vi "demo.vi"() -> ()   [LabVIEW 2017]
panel:
  out "z 4":dbl
  out "y 4":dbl
  out "x 4":dbl
  out "z 3":dbl
  out "y 3":dbl
  out "x 3":dbl
  out "z 2":dbl
  out "y 2":dbl
  out "x 2":dbl
  out "rv 2":dbl
  out "cx 3":dbl
  out "cy 3":dbl
  out "cz 3":dbl
  out "vx 3":dbl
  out "vy 3":dbl
  out "vz 3":dbl
  out "cx 2":dbl
  out "cy 2":dbl
  out "cz 2":dbl
  out "vx 2":dbl
  out "vy 2":dbl
  out "vz 2":dbl
  out "vz":dbl
  out "vy":dbl
  out "vx":dbl
  out "cz":dbl
  out "cy":dbl
  out "cx":dbl
  out "gap speed":dbl
  out "gap":dbl
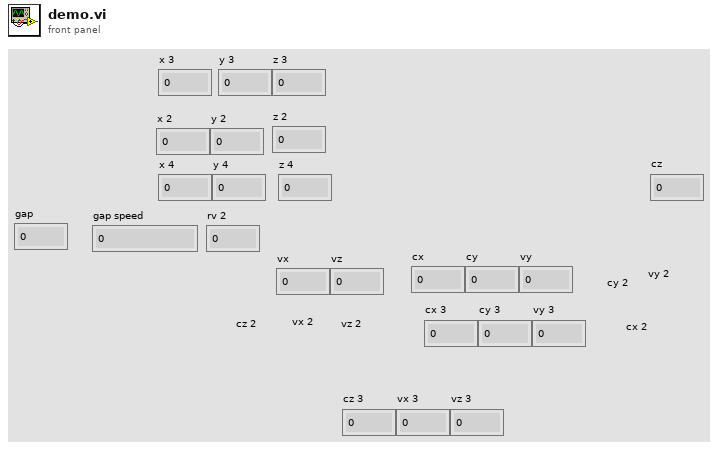
[diagram p1: front panel]
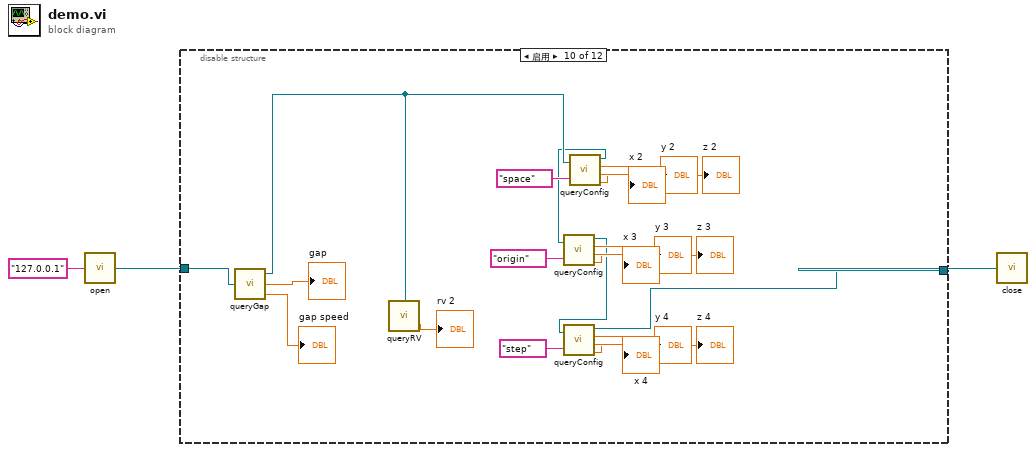
[diagram p0: block diagram]
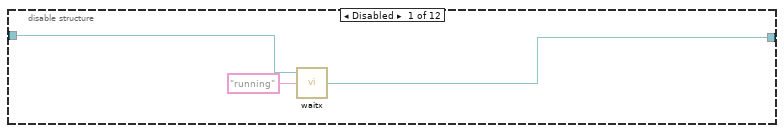
[diagram p2: hidden frame]
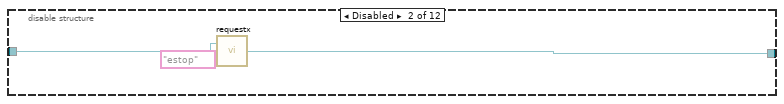
[diagram p3: hidden frame]
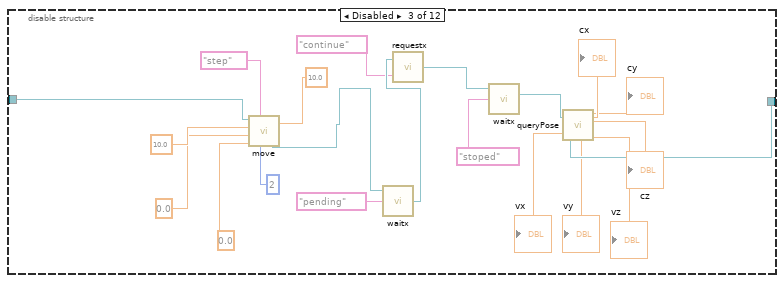
[diagram p4: hidden frame]
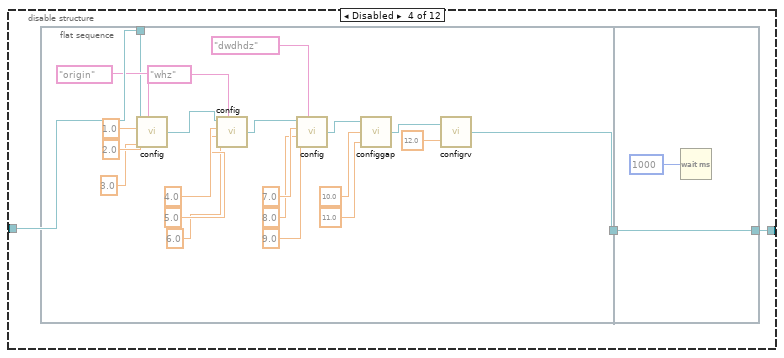
[diagram p5: hidden frame]
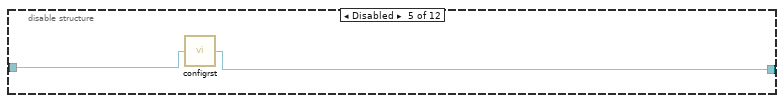
[diagram p6: hidden frame]
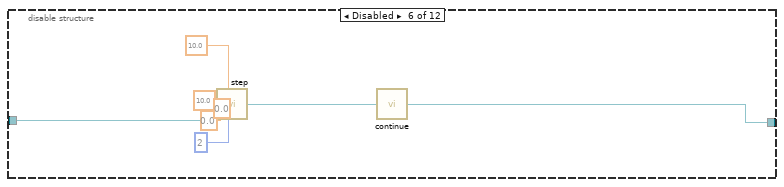
[diagram p7: hidden frame]
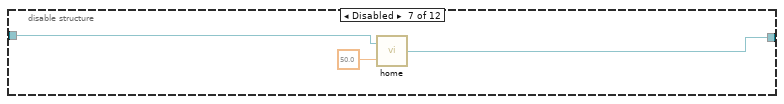
[diagram p8: hidden frame]
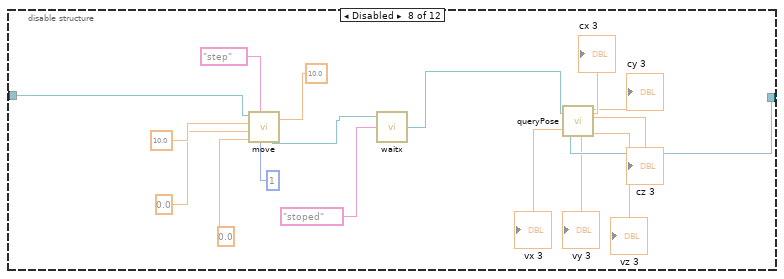
[diagram p9: hidden frame]
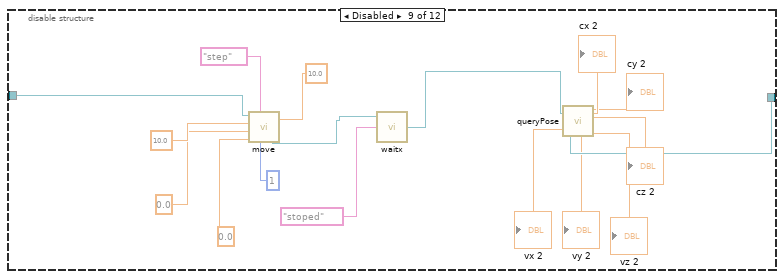
[diagram p10: hidden frame]
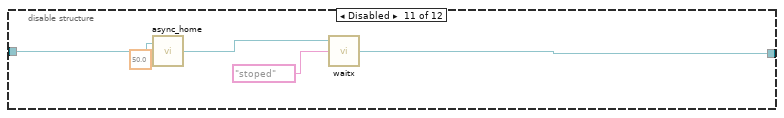
[diagram p11: hidden frame]
diagram:
  n1 = call "open.vi"("地址"="127.0.0.1") -> ("连接ID"=w2:refnum<k5>)
  n2 = disable-structure shown="启用" {
    disable-tunnel: w2 -> [w5 w9 w30 w33 w58 w66 w69 w86 w103 w123 w128 _]
    disable-tunnel: [w4 w7 w18 w32 w57 w59 w67 w73 w90 w104 w124 _] -> w1
    frame Disabled {
      n3 = call "waitx.vi"("String Value"="running", "连接ID"=w5) -> ("连接ID 2"=w4:refnum<k5>)  [unwired: 1 in]
    }
    frame Disabled {
      n4 = call "requestx.vi"("cmd"="estop" ("String"), "连接ID"=w9) -> ("连接ID输出"=w7:refnum<k5>)
    }
    frame Disabled {
      n5 = call "move.vi"("v"=10.0, "n"=2, "String"="step", "z"=0.0 ("zin"), "y"=0.0 ("yin"), "x"=10.0 ("xin"), "连接ID"=w30) -> ("连接ID输出"=w14:refnum<k5>)
      n6 = call "waitx.vi"("String Value"="pending", "连接ID"=w14) -> ("连接ID 2"=w12:refnum<k5>)  [unwired: 1 in]
      n7 = call "requestx.vi"("cmd"="continue" ("String"), "连接ID"=w12) -> ("连接ID输出"=w10:refnum<k5>)
      n8 = call "waitx.vi"("String Value"="stoped", "连接ID"=w10) -> ("连接ID 2"=w22:refnum<k5>)  [unwired: 1 in]
      n9 = call "queryPose.vi"("连接ID"=w22) -> ("连接ID输出"=w18:refnum<k5>, "x"=→"cx":dbl, "vx"=→"vx":dbl, "y"=→"cy":dbl, "z"=→"cz":dbl, "vy"=→"vy":dbl, "vz"=→"vz":dbl)
    }
    frame Disabled {
      n10 = flat-sequence {
        tunnel: w33 -> [w42]
        tunnel: [w37] -> w31
        tunnel: [w56] -> w32
        tunnel: w31 -> [w56]
        frame #0 {
          n11 = call "config.vi"("连接ID"=w42, "x"=1.0, "y"=2.0, "z"=3.0, "item"="origin" ("String")) -> ("连接ID输出"=w36:refnum<k5>)
          n12 = call "config.vi"("连接ID"=w36, "x"=4.0, "y"=5.0, "z"=6.0, "item"="whz" ("String")) -> ("连接ID输出"=w35:refnum<k5>)
          n13 = call "config.vi"("连接ID"=w35, "x"=7.0, "y"=8.0, "z"=9.0, "item"="dwdhdz" ("String")) -> ("连接ID输出"=w34:refnum<k5>)
          n14 = call "configgap.vi"("gapspeed"=11.0 ("y"), "gap"=10.0 ("x"), "连接ID"=w34) -> ("连接ID输出"=w39:refnum<k5>)
          n15 = call "configrv.vi"("rv"=12.0, "连接ID"=w39) -> ("连接ID输出"=w37:refnum<k5>)
        }
        frame #1 {
          n16 = Wait (ms)(milliseconds to wait=u32 1000 ("等待时间（毫秒）")) -> ()  [unwired: 1 out]
        }
      }
    }
    frame Disabled {
      n17 = call "configrst.vi"("连接ID"=w58) -> ("连接ID输出"=w57:refnum<k5>)
    }
    frame Disabled {
      n18 = call "step.vi"("n"=2, "v"=10.0, "z"=0.0, "y"=0.0, "x"=10.0, "连接ID"=w66) -> ("连接ID 2"=w62:refnum<k5>)
      n19 = call "continue.vi"("连接ID"=w62) -> ("连接ID 2"=w59:refnum<k5>)
    }
    frame Disabled {
      n20 = call "home.vi"("velocity"=50.0, "连接ID"=w69) -> ("连接ID 2"=w67:refnum<k5>)
    }
    frame Disabled {
      n21 = call "move.vi"("v"=10.0, "n"=1, "String"="step", "z"=0.0 ("zin"), "y"=0.0 ("yin"), "x"=10.0 ("xin"), "连接ID"=w86) -> ("连接ID输出"=w78:refnum<k5>)
      n22 = call "waitx.vi"("String Value"="stoped", "连接ID"=w78) -> ("连接ID 2"=w77:refnum<k5>)  [unwired: 1 in]
      n23 = call "queryPose.vi"("连接ID"=w77) -> ("连接ID输出"=w73:refnum<k5>, "x"=→"cx 3":dbl, "vx"=→"vx 3":dbl, "y"=→"cy 3":dbl, "z"=→"cz 3":dbl, "vy"=→"vy 3":dbl, "vz"=→"vz 3":dbl)
    }
    frame Disabled {
      n24 = call "move.vi"("v"=10.0, "n"=1, "String"="step", "z"=0.0 ("zin"), "y"=0.0 ("yin"), "x"=10.0 ("xin"), "连接ID"=w103) -> ("连接ID输出"=w95:refnum<k5>)
      n25 = call "waitx.vi"("String Value"="stoped", "连接ID"=w95) -> ("连接ID 2"=w94:refnum<k5>)  [unwired: 1 in]
      n26 = call "queryPose.vi"("连接ID"=w94) -> ("连接ID输出"=w90:refnum<k5>, "x"=→"cx 2":dbl, "vx"=→"vx 2":dbl, "y"=→"cy 2":dbl, "z"=→"cz 2":dbl, "vy"=→"vy 2":dbl, "vz"=→"vz 2":dbl)
    }
    frame Enabled {
      n27 = call "queryGap.vi"("连接ID"=w123) -> ("连接ID输出"=w115:refnum<k5>, "gap"=→"gap":dbl, "gap speed"=→"gap speed":dbl)
      n28 = call "queryRV.vi"("连接ID"=w115) -> ("rv"=→"rv 2":dbl)  [unwired: 1 out]
      n29 = call "queryConfig.vi"("连接ID"=w115, "item"="space" ("String")) -> ("连接ID输出"=w106:refnum<k5>, "x"=→"x 2":dbl, "y"=→"y 2":dbl, "z"=→"z 2":dbl)
      n30 = call "queryConfig.vi"("连接ID"=w106, "item"="origin" ("String")) -> ("连接ID输出"=w105:refnum<k5>, "x"=→"x 3":dbl, "y"=→"y 3":dbl, "z"=→"z 3":dbl)
      n31 = call "queryConfig.vi"("连接ID"=w105, "item"="step" ("String")) -> ("连接ID输出"=w104:refnum<k5>, "x"=→"x 4":dbl, "y"=→"y 4":dbl, "z"=→"z 4":dbl)
    }
    frame Disabled {
      n32 = call "async_home.vi"("velocity"=50.0, "连接ID"=w128) -> ("连接ID输出"=w125:refnum<k5>)
      n33 = call "waitx.vi"("String Value"="stoped", "连接ID"=w125) -> ("连接ID 2"=w124:refnum<k5>)  [unwired: 1 in]
    }
    frame Disabled {
    }
  }
  n34 = call "close.vi"("连接ID"=w1) -> ()
